vi "velosterpaser.vi"(8 "x":dbl) -> ()   [LabVIEW 2015]
uses:
  G_VEH.vi
  G_NAV.vi
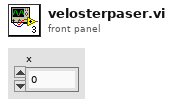
[diagram p1: front panel]
types:
  T1 = enum16{"big-endian, network order", "native, host order", "little-endian"}
  T2 = cluster{"GPSTime":dbl, "accel[0]":sgl, "accel[1]":sgl, "accel[2]":sgl, "pqr[0]":sgl, "pqr[1]":sgl, "pqr[2]":sgl, "llh[0]":dbl, "llh[1]":dbl, "llh[2]":dbl, "vel_ned[0]":sgl, "vel_ned[1]":sgl, "vel_ned[2]":sgl, "attitude[0]":sgl, "attitude[1]":sgl, "attitude[2]":sgl, "vel_bxyz[0]":sgl, "vel_bxyz[1]":sgl, "vel_bxyz[2]":sgl, "lcc[0]":sgl, "lcc[1]":sgl, "lcc[2]":sgl, "CovKalman[0]":sgl, "CovKalman[1]":sgl, "CovKalman[2]":sgl, "CovKalman[3]":sgl, "CovKalman[4]":sgl, "CovKalman[5]":sgl, "llh_GPS[0]":sgl, "llh_GPS[1]":sgl, "llh_GPS[2]":sgl, "vel_GPS[0]":sgl, "vel_GPS[1]":sgl, "vel_GPS[2]":sgl, "heading_Magnetic":sgl, "heading_GPS":sgl, "GPSStatus":u16, "FailureCode":u16, "DataChecksum":u16}
  T3 = cluster{"sop1":u8, "sop2":u8, "sop3":u8, "header_length":u8, "number":u16, "type":u8, "port_address":u8, "length":u16, "sequence":u16, "idle":u8, "gps_stat":u8, "gps_week":u16, "millisecs":u32, "status":u32, "crc":u16, "version":u16}
  T4 = cluster{"sol_stat":u32, "pos_type":u32, "lat":dbl, "lon":dbl, "hgt":dbl, "und":sgl, "datum_id":i32, "latdev":sgl, "londev":sgl, "hgtdev":sgl, "ref_station_id 0":i8, "ref_station_id 1":i8, "ref_station_id 2":i8, "ref_station_id 3":i8, "lag":sgl, "age":sgl, "sats":u8, "gps_l1_ranges":u8, "gps_l1_mask_ranges":u8, "gps_l2_mask_ranges":u8, "reserved":i8, "ext_sol_stat":u8, "reserved2":u8, "sig_mask":u8}
  T5 = cluster{"Steer_input":dbl, "Steer_output":dbl, "VS_des":dbl, "VS_can":dbl, "heading":dbl, "auto":bool, "run":bool, "x":dbl, "y":dbl}
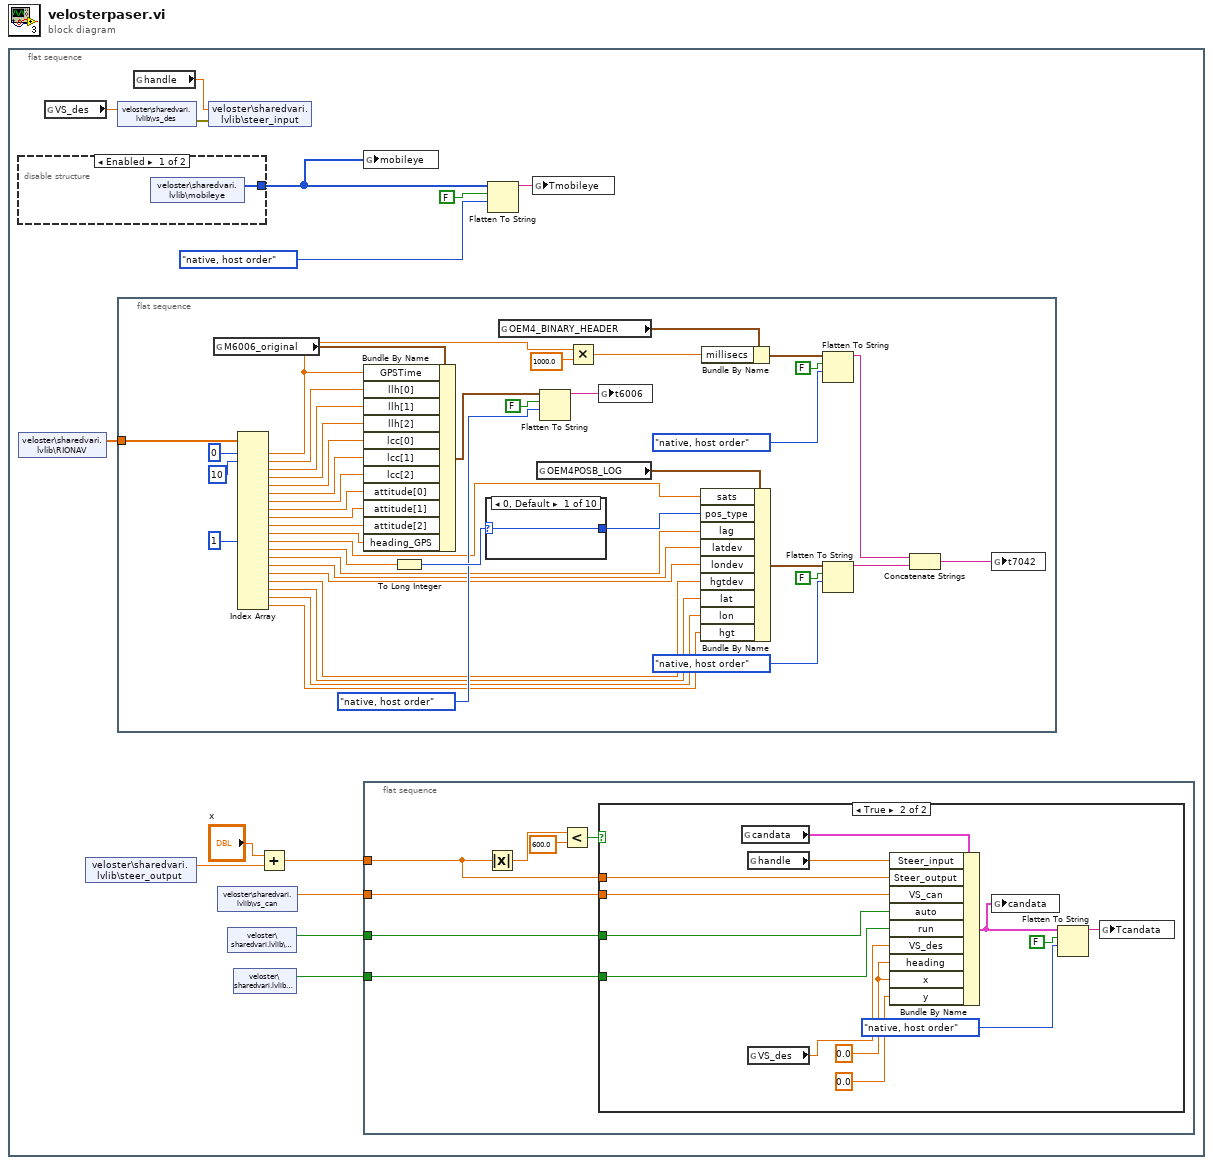
[diagram p0: block diagram]
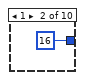
[diagram p3: hidden frame]
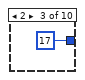
[diagram p4: hidden frame]
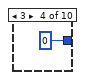
[diagram p5: hidden frame]
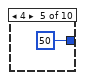
[diagram p6: hidden frame]
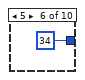
[diagram p7: hidden frame]
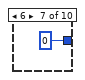
[diagram p8: hidden frame]
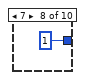
[diagram p9: hidden frame]
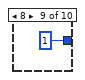
[diagram p10: hidden frame]
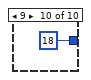
[diagram p11: hidden frame]
diagram:
  n1 = flat-sequence {
    frame #0 {
      n2 = disable-structure shown="Enabled" {
        disable-tunnel: [w15 _] -> w5
        frame Enabled {
          n3 = shared-variable "veloster\\sharedvari.lvlib\\mobileye"() -> (w15:u8[])  [unwired: 1 in, 1 out]
        }
        frame Disabled {
        }
      }
      n4 = shared-variable "veloster\\sharedvari.lvlib\\RIONAV"() -> (w11:dbl[])  [unwired: 1 in, 1 out]
      n5 = global read "G_VEH.vi" "VS_des"() -> (w9:dbl)
      n6 = shared-variable "veloster\\sharedvari.lvlib\\steer_output"() -> (w3:dbl)  [unwired: 1 in, 1 out]
      n7 = shared-variable "veloster\\sharedvari.lvlib\\vs_des"(w9) -> (error out=w8:errorcluster)  [unwired: 1 in]
      n8 = flat-sequence {
        tunnel: w11 -> [w18]
        frame #0 {
          n9 = global read "G_NAV.vi" "M6006_original"() -> (w58:T2)
          n10 = Index Array(array=w18, index #1=0 ("index"), index #2=10 ("index"), index #12=1 ("index")) -> (element #1=w47:dbl, element #2=w56:dbl, element #3=w55:dbl, element #4=w54:dbl, element #5=w17:dbl, element #6=w20:dbl, element #7=w53:dbl, element #8=w16:dbl, element #9=w52:dbl, element #10=w19:dbl, element #11=w23:dbl, element #12=w25:dbl, element #13=w26:dbl, element #14=w27:dbl, element #15=w28:dbl, element #16=w29:dbl, element #17=w30:dbl, element #18=w22:dbl, element #19=w21:dbl, element #20=w31:dbl)  [unwired: 17 in]
          n11 = Bundle By Name(cluster=w58, "GPSTime"=w47, "llh[0]"=w56, "llh[1]"=w55, "llh[2]"=w54, "lcc[0]"=w17, "lcc[1]"=w20, "lcc[2]"=w53, "attitude[0]"=w16, "attitude[1]"=w52, "attitude[2]"=w19, "heading_GPS"=w23) -> (w44:T2)
          n12 = To Long Integer(number=w26) -> (32bit integer=w50:i32)
          n13 = case shown="0, Default" w50 {
            selector: w50 -> [w60 _ _ _ _ _ _ _ _ _]
            tunnel: [w60 16 17 0 50 34 0 1 1 18] -> w49
            frame 0, Default {
            }
            frame 1 {
            }
            frame 2 {
            }
            frame 3 {
            }
            frame 4 {
            }
            frame 5 {
            }
            frame 6 {
            }
            frame 7 {
            }
            frame 8 {
            }
            frame 9 {
            }
          }
          n14 = global read "G_NAV.vi" "OEM4_BINARY_HEADER"() -> (w48:T3)
          n15 = global read "G_NAV.vi" "OEM4POSB_LOG"() -> (w51:T4)
          n16 = Flatten To String(anything=w44, prepend array or string size? (T)=FALSE, byte order (0:big-endian, network order)=T1."native, host order") -> (data string=w41:string)  [unwired: 1 in, 2 out]
          n17 = Multiply(x=w47, y=1000.0) -> (x*y=w45:dbl)
          n18 = global write "G_NAV.vi" "t6006"(w41) -> ()
          n19 = Bundle By Name(cluster=w51, "sats"=w25, "pos_type"=w49, "lag"=w27, "latdev"=w28, "londev"=w29, "hgtdev"=w30, "lat"=w22, "lon"=w21, "hgt"=w31) -> (w35:T4)
          n20 = Bundle By Name(cluster=w48, "millisecs"=w45) -> (w39:T3)
          n21 = Flatten To String(anything=w39, prepend array or string size? (T)=FALSE, byte order (0:big-endian, network order)=T1."native, host order") -> (data string=w34:string)  [unwired: 1 in, 2 out]
          n22 = Flatten To String(anything=w35, prepend array or string size? (T)=FALSE, byte order (0:big-endian, network order)=T1."native, host order") -> (data string=w33:string)  [unwired: 1 in, 2 out]
          n23 = Concatenate Strings(w34, w33) -> (w32:string)
          n24 = global write "G_NAV.vi" "t7042"(w32) -> ()
        }
      }
      n25 = global read "G_VEH.vi" "handle"() -> (w10:dbl)
      n26 = shared-variable "veloster\\sharedvari.lvlib\\steer_input"(w10, error in=w8) -> ()  [unwired: 1 out]
      n27 = shared-variable "veloster\\sharedvari.lvlib\\vs_can"() -> (w14:dbl)  [unwired: 1 in, 1 out]
      n28 = shared-variable "veloster\\sharedvari.lvlib\\auto"() -> (w12:bool)  [unwired: 1 in, 1 out]
      n29 = shared-variable "veloster\\sharedvari.lvlib\\run"() -> (w13:bool)  [unwired: 1 in, 1 out]
      n30 = Add(x="x", y=w3) -> (x+y=w1:dbl)
      n31 = global write "G_VEH.vi" "mobileye"(w5) -> ()
      n32 = flat-sequence {
        tunnel: w14 -> [w73]
        tunnel: w13 -> [w72]
        tunnel: w12 -> [w71]
        tunnel: w1 -> [w70]
        frame #0 {
          n33 = Absolute Value(x=w70) -> (abs(x)=w76:dbl)
          n34 = Less?(x=w76, y=600.0) -> (x < y?=w74:bool)
          n35 = case shown="True" w74 {
            tunnel: w70 -> [_ w89]
            tunnel: w71 -> [_ w82]
            tunnel: w72 -> [_ w81]
            tunnel: w73 -> [_ w83]
            frame False {
            }
            frame True {
              w78 = 0.0 ("x")
              n36 = global read "G_VEH.vi" "candata"() -> (w84:T5)
              n37 = global read "G_VEH.vi" "handle"() -> (w77:dbl)
              n38 = global read "G_VEH.vi" "VS_des"() -> (w80:dbl)
              n39 = Bundle By Name(cluster=w84, "Steer_input"=w77, "Steer_output"=w89, "VS_can"=w83, "auto"=w82, "run"=w81, "VS_des"=w80, "heading"=w78, "x"=w78, "y"=0.0) -> (w88:T5)
              n40 = global write "G_VEH.vi" "candata"(w88) -> ()
              n41 = Flatten To String(anything=w88, prepend array or string size? (T)=FALSE, byte order (0:big-endian, network order)=T1."native, host order") -> (data string=w85:string)  [unwired: 1 in, 2 out]
              n42 = global write "G_VEH.vi" "Tcandata"(w85) -> ()
            }
          }
        }
      }
      n43 = Flatten To String(anything=w5, prepend array or string size? (T)=FALSE, byte order (0:big-endian, network order)=T1."native, host order") -> (data string=w7:string)  [unwired: 1 in, 2 out]
      n44 = global write "G_VEH.vi" "Tmobileye"(w7) -> ()
    }
  }
